vi "Vector_convert.vi"(11 "x,y":cluster{dbl, dbl}) -> (2 "angle":dbl, 3 "mag":dbl)   [LabVIEW 2024]
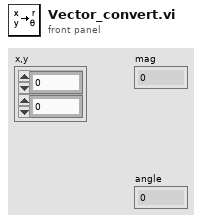
[diagram p1: front panel]
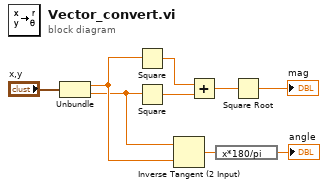
[diagram p0: block diagram]
diagram:
  n1 = Unbundle("x,y") -> (w6:dbl, w5:dbl)
  n2 = Square(x=w6) -> (x^2=w2:dbl)
  n3 = Square(x=w5) -> (x^2=w4:dbl)
  n4 = Inverse Tangent (2 Input)(1:w6, 2:w5) -> (0:w7:dbl)
  n5 = Add(x=w2, y=w4) -> (x+y=w3:dbl)
  n6 = expression code="x*180/pi"(w7) -> (→"angle":dbl)
  n7 = Square Root(x=w3) -> (sqrt(x)=→"mag":dbl)
